vi "testServo.vi"() -> ()   [LabVIEW 2011]
uses:
  GlobalSerial.vi
panel:
  out "error out 2":errorcluster
  out "serial status":u32(colorbox)
  in  "speed":u8
  in  "channel":u8
  out "*(type *) &x":u8[](array[numeric])
  out "concatenated string":string
  in  "servo position":u16(knob)=260 min=260 max=1150 step=1 scale=260.0..1150.0
  in  "stop":bool
  in  "VISA resource name":refnum<visa-resource-name>="COM3"
  out "error out":errorcluster
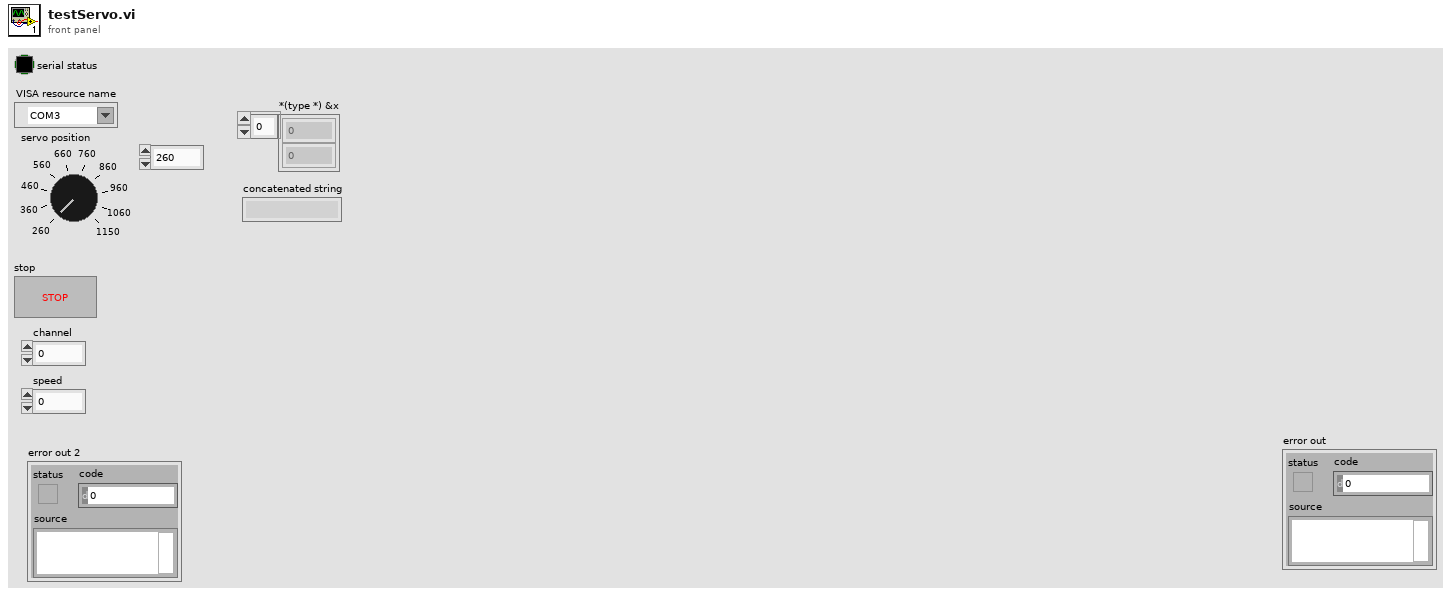
[diagram p1: front panel]
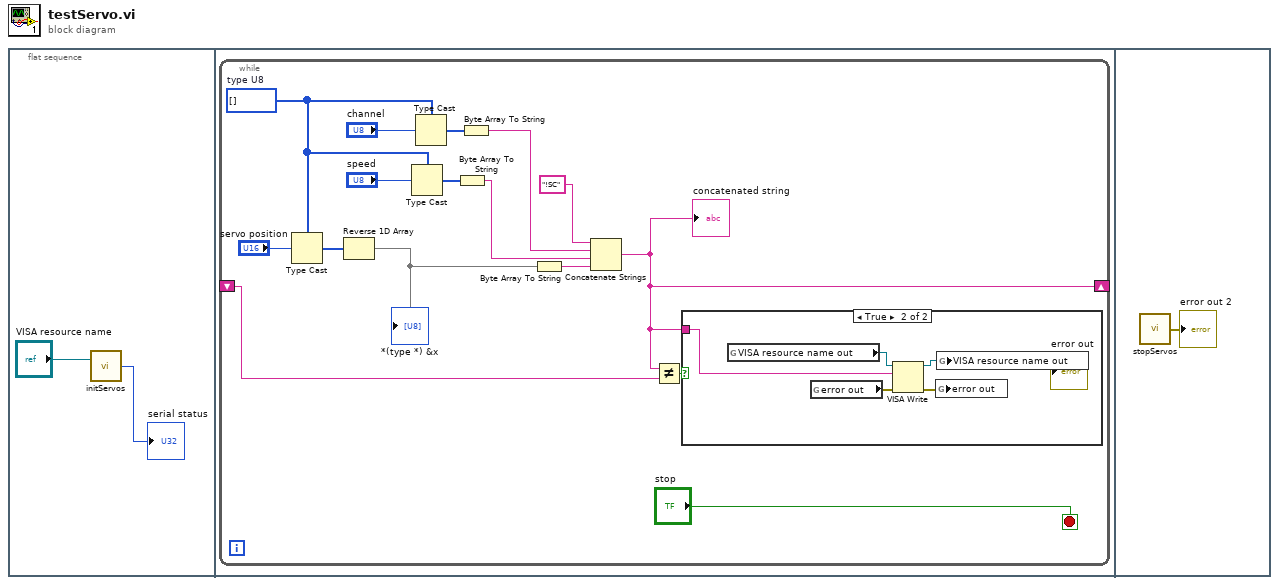
[diagram p0: block diagram]
diagram:
  n1 = flat-sequence {
    frame #0 {
      n2 = call "initServos.vi"("VISA resource name"="VISA resource name") -> ("serial status"=→"serial status":u32)
    }
    frame #1 {
      n3 = while {
        shift-right: [w10] -> _
        shift-left: _ -> [w12]
        stop <- "stop" stop-if-true
        w6 = u8[] []  # type U8
        n4 = Type Cast(type=w6, x="servo position") -> (*(type *) &x=w13:u8[])
        n5 = Reverse 1D Array(array=w13) -> (reversed array=w14:u8[])
        "*(type *) &x" <- w14
        n6 = Type Cast(type=w6, x="speed") -> (*(type *) &x=w5:u8[])
        n7 = Type Cast(type=w6, x="channel") -> (*(type *) &x=w8:u8[])
        n8 = Byte Array To String(unsigned byte array=w5) -> (string=w4:string)
        n9 = Byte Array To String(unsigned byte array=w8) -> (string=w9:string)
        n10 = Byte Array To String(unsigned byte array=w14) -> (string=w15:string)
        n11 = Concatenate Strings("!SC" ("string"), w9, w4, w15) -> (w10:string)
        "concatenated string" <- w10
        n12 = Not Equal?(x=w10, y=w12) -> (x != y?=w11:bool)
        n13 = case shown="True" w11 {
          tunnel: w10 -> [_ w23]
          frame False {
          }
          frame True {
            n14 = global read "GlobalSerial.vi" "VISA resource name out"() -> (w19:refnum<visa-resource-name>)
            n15 = global read "GlobalSerial.vi" "error out"() -> (w21:errorcluster)
            n16 = VISA Write(VISA resource name=w19, write buffer=w23, error in (no error)=w21) -> (VISA resource name out=w20:refnum<visa-resource-name>, error out=w22:errorcluster)  [unwired: 1 out]
            n17 = global write "GlobalSerial.vi" "error out"(w22) -> ()
            n18 = global write "GlobalSerial.vi" "VISA resource name out"(w20) -> ()
          }
        }
      }
    }
    frame #2 {
      n19 = call "stopServos.vi"() -> ("error out"=→"error out 2":errorcluster)  [unwired: 2 in]
    }
  }
